vi "Block Diagram While Loop Scripting.vi"() -> ()   [LabVIEW 2014]
uses:
  <vilib>/Utility/traverseref.llb/TRef TravTarget.ctl
  <vilib>/Utility/traverseref.llb/VI Scripting - Traverse.lvlib
panel:
  out "# of Refs":i32
  out "error IO":errorcluster
  out "String":string
  in  "error in":errorcluster
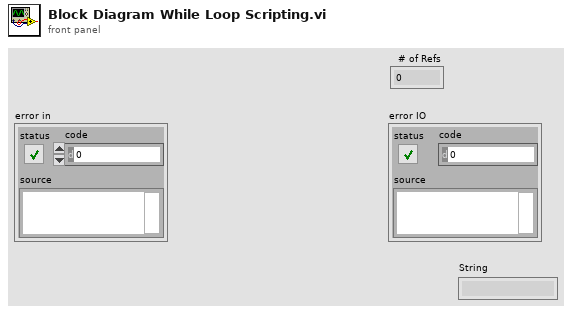
[diagram p1: front panel]
types:
  T1 = typedef "TRef TravTarget.ctl" = enum16{"FP", "BD", "Other"}
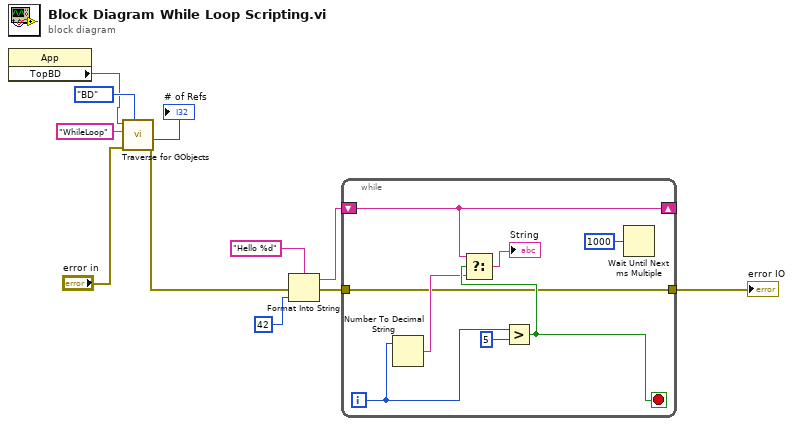
[diagram p0: block diagram]
diagram:
  n1 = property class="App"() -> ("TopBD"=w3:refnum<vi>)  [unwired: 2 in, 2 out]
  n2 = call <vilib>:"Traverse for GObjects.vi"("Traverse Target"=TRef_TravTarget."BD", "error in (no error)"="error in", "Class Name"="WhileLoop", "VI Refnum"=w3) -> ("error out"=w2:errorcluster, "# of Refs"=→"# of Refs":i32)  [unwired: 4 in, 2 out]
  n3 = Format Into String(format string="Hello %d", error in=w2, 42) -> (resulting string=w8:string, error out=w9:errorcluster)  [unwired: 1 in]
  n4 = while {
    tunnel: w9 -> [w12]
    shift-right: [w15] -> _
    shift-left: w8 -> [w15]
    tunnel: [w12] -> w7
    i -> [w17]
    stop <- w18 stop-if-true
    n5 = Number To Decimal String(number=w17) -> (decimal integer string=w16:string)  [unwired: 1 in]
    n6 = Greater?(x=w17, y=5) -> (0:w18:bool)
    n7 = Select(t=w15, s=w18, f=w16) -> (s? t:f=→"String":string)
    n8 = Wait Until Next ms Multiple(millisecond multiple=u32 1000) -> ()  [unwired: 1 out]
  }
  "error IO" <- w7
